vi "Merge_PKYK_Imgs.vi"(1 "Img. In":picture[](array[picture])) -> (0 "PKYK 1":picture)   [LabVIEW 2020]
uses:
  <vilib>/picture/picture.llb/Draw True-Color Pixmap.vi
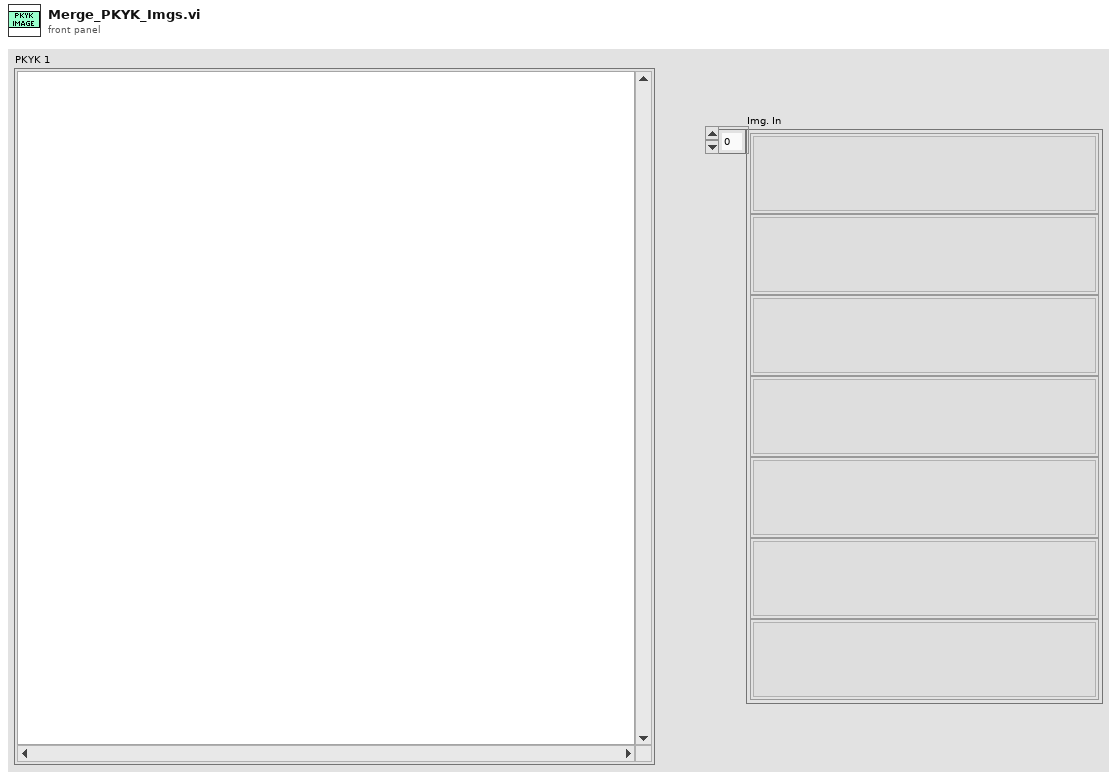
[diagram p1: front panel]
types:
  T1 = cluster{"left":i16, "top":i16, "right":i16, "bottom":i16}
  T2 = typedef "imagedata.ctl" = cluster{"image type":i32, "image depth":i32, "image":u8[], "mask":u8[], "colors":u32[], "Rectangle":cluster{"left":i16, "top":i16, "right":i16, "bottom":i16}}
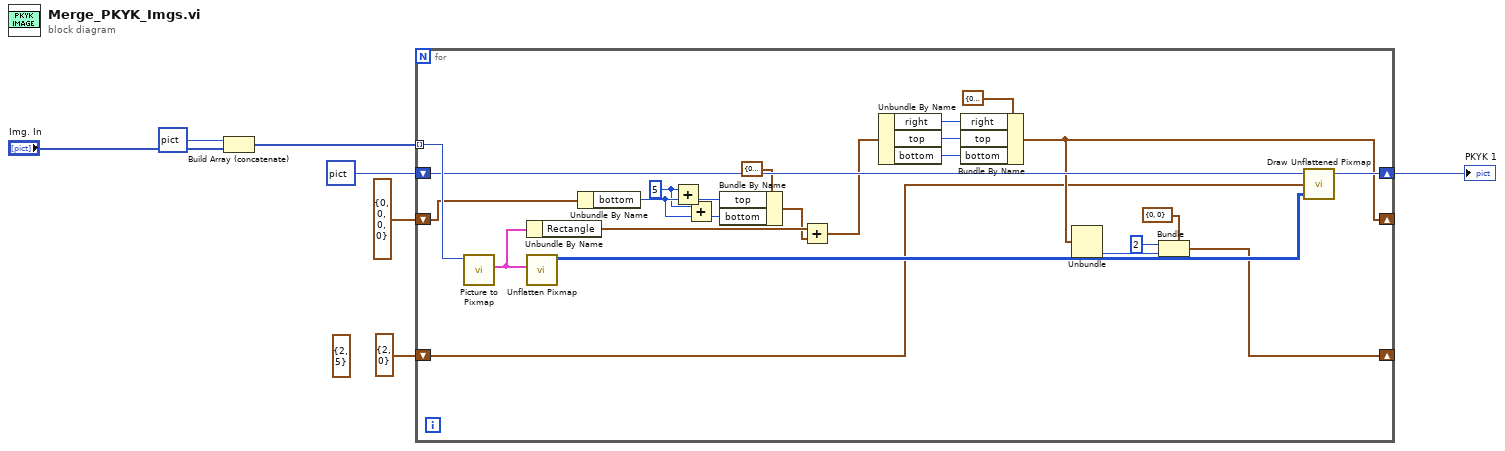
[diagram p0: block diagram]
diagram:
  (unwired) cluster{"x":i16, "y":i16} {"x"=2, "y"=5} ("point")
  n1 = Build Array (concatenate)(picture bytes[31926] ("PKYK"), "Img. In") -> (w6:picture[])
  n2 = for {
    tunnel: w6 -> [w30] mode=indexing
    shift-right: [w28] -> w4
    shift-left: picture data[5B] ("PKYK") -> [w29]
    shift-right: [w19] -> _
    shift-left: T1 {"left"=0, "top"=0, "right"=0, "bottom"=0} ("Rectangle") -> [w22]
    shift-right: [w13] -> _
    shift-left: cluster{"x":i16, "y":i16} {"x"=2, "y"=0} ("point") -> [w15]
    w8 = i16 5 ("x")
    n3 = call <vilib>:"Picture to Pixmap.vi"("picture"=w30) -> ("image data"=w25:T2)  [unwired: 9 in, 1 out]
    n4 = Unbundle By Name(w25) -> ("Rectangle"=w24:T1)
    n5 = call <vilib>:"Unflatten Pixmap.vi"("image data"=w25) -> ("24-bit pixmap"=w31:u32[][])  [unwired: 4 in, 6 out]
    n6 = Unbundle By Name(w22) -> ("bottom"=w17:i16)
    n7 = Add(x=w8, y=w17) -> (x+y=w10:i16)
    n8 = Add(x=w8, y=w17) -> (x+y=w9:i16)
    n9 = Bundle By Name(cluster=T1 {"left"=0, "top"=0, "right"=0, "bottom"=0} ("Rectangle"), "top"=w10, "bottom"=w9) -> (w16:T1)
    n10 = Add(x=w24, y=w16) -> (x+y=w23:T1)
    n11 = Unbundle By Name(w23) -> ("right"=w14:i16, "top"=w26:i16, "bottom"=w27:i16)
    n12 = Bundle By Name(cluster=T1 {"left"=0, "top"=0, "right"=0, "bottom"=0} ("Rectangle"), "right"=w14, "top"=w26, "bottom"=w27) -> (w19:T1)
    n13 = Unbundle(w19) -> ("bottom"=w11:i16)  [unwired: 3 out]
    n14 = Bundle(cluster=cluster{"x":i16, "y":i16} {"x"=0, "y"=0} ("point"), "x"=i16 2, "y"=w11) -> (w13:cluster{"x":i16, "y":i16})
    n15 = call-poly <vilib>:"Draw Unflattened Pixmap.vi"("picture"=w29, "top left point(0, 0)"=w15, "data (RGB format)"=w31) -> ("new picture"=w28:picture)  [unwired: 6 in]
  }
  "PKYK 1" <- w4
